vi "CheckTemplateChange.vi"(8 "Template #":i8, 9 "Template":string, 10 "Settings In":T1={"Name of test"="", "Date"=timestamp(0 s since 1904-01-01), "Location"="", "Template"="", "Soundcard"="", "resolution"=0, "Sampling rate"=0, "Ch1 Gain "=0.0, "Ch2 Gain"=0.0, "Sample time (s)"=0.0, "Pre-trigger (s)"=0.0, "Hammer Threshold"=0.0, "Positions"=0, "Taps/Position"=0, "Set Names"="", "Freq resolution"=0.0, "Hammer cutoff"=0.0, "Mic cutoff"=0.0, "Double bounce "=0.0, "Hammer Cal"=0.0, "dB Offset"=0.0, "Accel Cal"=0.0, "Vibrometer Cal"=0.0, "Mic Cal"=0.0, "Output"=0, "Voltage Cal"=0.0, "Vibrometer Port"="", "Range"=0, "High Pass"=0, "Bandwidth"=0, "X Range"=[], "Y Range"=[], "dB Spread"=0.0, "Trigger"=0, "Ch_1"=0, "Ch_2"=0, "flip?"=FALSE, "60Hz"=FALSE, "Time offset"=0.0, "Piezo Cal"=1.0, "Default Notes"=""} {"Ch_2" min=1 step=1; "Ch_1" min=1 max=100 step=1; "Trigger" items=["Hammer (force)", "Self-tap", "Spacebar"]; "Bandwidth" items=["1 kHz"=1, "5 kHz"=5, "10 kHz"=10, "25 kHz"=25, "50 kHz"=50, "100 kHz"=100]; "High Pass" items=["Off", "13 Hz", "104 Hz"]; "Range" items=["10 mm/s"=1, "20 mm/s"=2, "50 mm/s"=5, "100 mm/s"=10, "200 mm/s"=20, "500 mm/s"=50, "1 m/s"=100, "2 m/s"=200]; "Output" items=["Accelerometer", "Speed (from acceleration)", "Microphone", "Vibrometer", "Piezo"]; "Voltage Cal" format="%#_13g"; "Ch2 Gain" format="%#_13g"; "Ch1 Gain" format="%#_13g"; "Double bounce" min=0.0; "Mic cutoff" min=0.0 format="%#_4g"; "Hammer cutoff" min=0.0 format="%#_4g"; "Freq resolution" min=0.0; "Pre-trigger (s)" format="%#_13g"; "Date" format="%<%H:%M\n%d/%m/%y>T"; "resolution" items=["16 bit"=16, "24 bit"=24, "32 bit"=32]; "Sampling rate" items=["22050 samp/s"=22050, "44100 samp/s"=44100, "48000 samp/s"=48000]}, 11 "Path To Instrument Folder":path) -> (2 "Template":u16, 3 "Settings  Out":T1={"Name of test"="", "Date"=timestamp(0 s since 1904-01-01), "Location"="", "Template"="", "Soundcard"="", "resolution"=0, "Sampling rate"=0, "Ch1 Gain "=0.0, "Ch2 Gain"=0.0, "Sample time (s)"=0.0, "Pre-trigger (s)"=0.0, "Hammer Threshold"=0.0, "Positions"=0, "Taps/Position"=0, "Set Names"="", "Freq resolution"=0.0, "Hammer cutoff"=0.0, "Mic cutoff"=0.0, "Double bounce "=0.0, "Hammer Cal"=0.0, "dB Offset"=0.0, "Accel Cal"=0.0, "Vibrometer Cal"=0.0, "Mic Cal"=0.0, "Output"=0, "Voltage Cal"=0.0, "Vibrometer Port"="", "Range"=0, "High Pass"=0, "Bandwidth"=0, "X Range"=[], "Y Range"=[], "dB Spread"=0.0, "Trigger"=0, "Ch_1"=0, "Ch_2"=0, "flip?"=FALSE, "60Hz"=FALSE, "Time offset"=0.0, "Piezo Cal"=1.0, "Default Notes"=""} {"Ch_2" min=1 step=1; "Ch_1" min=1 max=100 step=1; "Trigger" items=["Hammer (force)", "Self-tap", "Spacebar"]; "Bandwidth" items=["1 kHz"=1, "5 kHz"=5, "10 kHz"=10, "25 kHz"=25, "50 kHz"=50, "100 kHz"=100]; "High Pass" items=["Off", "13 Hz", "104 Hz"]; "Range" items=["10 mm/s"=1, "20 mm/s"=2, "50 mm/s"=5, "100 mm/s"=10, "200 mm/s"=20, "500 mm/s"=50, "1 m/s"=100, "2 m/s"=200]; "Output" items=["Accelerometer", "Speed (from acceleration)", "Microphone", "Vibrometer", "Piezo"]; "Voltage Cal" format="%#_13g"; "Ch2 Gain" format="%#_13g"; "Ch1 Gain" format="%#_13g"; "Double bounce" min=0.0; "Mic cutoff" min=0.0 format="%#_4g"; "Hammer cutoff" min=0.0 format="%#_4g"; "Freq resolution" min=0.0; "Pre-trigger (s)" format="%#_13g"; "Date" format="%<%H:%M\n%d/%m/%y>T"; "resolution" items=["16 bit"=16, "24 bit"=24, "32 bit"=32]; "Sampling rate" items=["22050 samp/s"=22050, "44100 samp/s"=44100, "48000 samp/s"=48000]})   [LabVIEW 2022 SP3]
uses:
  PreferencesControl.ctl
panel:
  # "Hz"
  # "dB"
  # "dB"
  # "sec"
  # "sec"
  # "mV/Pa"
  # "mV/m/s2"
  # "mV/mm/s"
  # "V/N"
  # "sec"
  # "sec"
  # "mV/N"
  # "a.u."
  # "a.u."
  # "sec"
  # "Hz"
  # "dB"
  # "dB"
  # "sec"
  # "sec"
  # "mV/Pa"
  # "mV/m/s2"
  # "mV/mm/s"
  # "V/N"
  # "sec"
  # "sec"
  # "mV/N"
  # "a.u."
  # "a.u."
  # "sec"
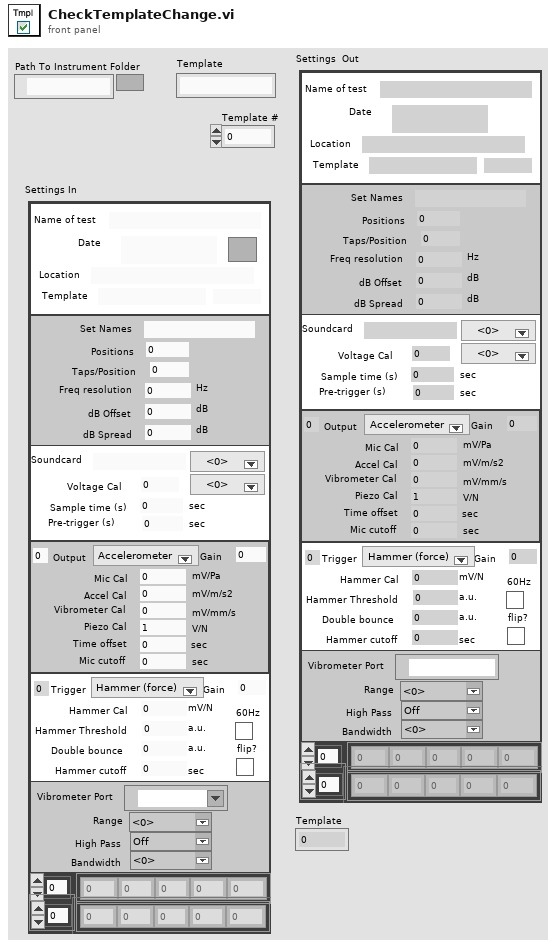
[diagram p1: front panel]
types:
  T1 = typedef "PreferencesControl.ctl" = cluster{"Name of test":string, "Date":timestamp, "Location":string, "Template":string, "Soundcard":string, "resolution":u16, "Sampling rate":u16, "Ch1 Gain ":dbl, "Ch2 Gain":dbl, "Sample time (s)":dbl, "Pre-trigger (s)":dbl, "Hammer Threshold":dbl, "Positions":i16, "Taps/Position":i16, "Set Names":string, "Freq resolution":dbl, "Hammer cutoff":dbl, "Mic cutoff":dbl, "Double bounce ":dbl, "Hammer Cal":dbl, "dB Offset":dbl, "Accel Cal":dbl, "Vibrometer Cal":dbl, "Mic Cal":dbl, "Output":u16, "Voltage Cal":dbl, "Vibrometer Port":refnum<visa-resource-name>, "Range":u16, "High Pass":u16, "Bandwidth":u16, "X Range":cluster{"Minimum":dbl, "Maximum":dbl, "Increment":dbl, "Minor Increment":dbl, "Start":dbl}[], "Y Range":cluster{"Minimum":dbl, "Maximum":dbl, "Increment":dbl, "Minor Increment":dbl, "Start":dbl}[], "dB Spread":dbl, "Trigger":u16, "Ch_1":u8, "Ch_2":u8, "flip?":bool, "60Hz":bool, "Time offset":dbl, "Piezo Cal":dbl, "Default Notes":string}
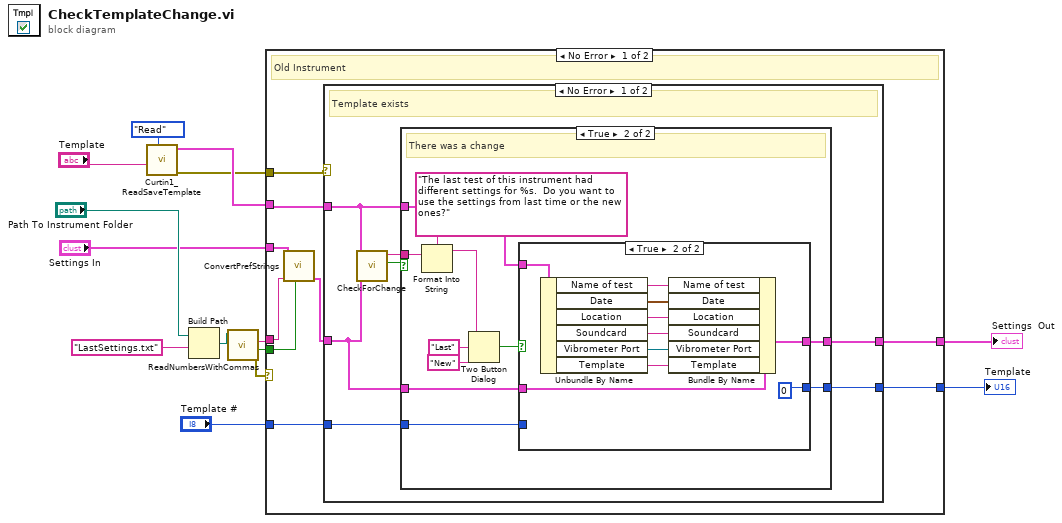
[diagram p0: block diagram]
diagram:
  n1 = call "Curtin1_ReadSaveTemplate.vi"("Task"=enum16{"Save", "Read", "List"}."Read", "Template"="Template") -> ("error out"=w5:errorcluster, "Settings out"=w6:T1)  [unwired: 6 in, 2 out]
  n2 = Build Path(base path="Path To Instrument Folder", name or relative path="LastSettings.txt") -> (appended path=w4:path)
  n3 = call "ReadNumbersWithCommas.vi"("file (use dialog)"=w4) -> ("error out"=w3:errorcluster, "comma?"=w1:bool, "text"=w2:string)  [unwired: 7 in, 1 out]
  n4 = case shown="No Error" w3 {
    tunnel: w2 -> [w23 _]
    tunnel: "Settings In" -> [w22 _]
    tunnel: [w19 w58] -> w11
    tunnel: w6 -> [w18 w59]
    tunnel: "Template #" -> [w17 w58]
    tunnel: [w21 w59] -> w8
    tunnel: w5 -> [w16 _]
    tunnel: w1 -> [w15 _]
    frame No Error {
      # "Old Instrument"
      n5 = call "ConvertPrefStrings.vi"("Comma?"=w15, "String In"=w23, "Settings"=w22) -> ("Settings"=w20:T1)  [unwired: 7 in, 1 out]
      n6 = case shown="No Error" w16 {
        tunnel: [w28 w56] -> w21
        tunnel: w20 -> [w27 w56]
        tunnel: [w26 w57] -> w19
        tunnel: w18 -> [w25 _]
        tunnel: w17 -> [w24 w57]
        frame No Error {
          # "Template exists"
          n7 = call "CheckForChange.vi"("Original Settings"=w27, "Current Settings"=w25) -> ("change?"=w30:bool, "list of changes"=w29:string)  [unwired: 8 in]
          n8 = case shown="True" w30 {
            tunnel: w29 -> [_ w42]
            tunnel: [w32 w37] -> w28
            tunnel: w27 -> [_ w36]
            tunnel: [w31 w35] -> w26
            tunnel: w25 -> [w32 w34]
            tunnel: w24 -> [w31 w33]
            frame False {
              # "Same settings"
            }
            frame True {
              # "There was a change"
              n9 = Format Into String(format string="The last test of this instrument had different settings for %s.  Do you want to use the settings from last time or the new ones?", w42) -> (resulting string=w41:string)  [unwired: 2 in, 1 out]
              n10 = Two Button Dialog(message=w41, 1:"New" ("F button name (\"Cancel\")"), 2:"Last" ("T button name (\"OK\")")) -> (T button?=w38:bool)
              n11 = case shown="True" w38 {
                tunnel: [w45 w47] -> w37
                tunnel: w36 -> [_ w48]
                tunnel: [w44 0] -> w35
                tunnel: w34 -> [w45 w49]
                tunnel: w33 -> [w44 _]
                frame False {
                }
                frame True {
                  n12 = Unbundle By Name(w49) -> ("Name of test"=w54:string, "Date"=w53:timestamp, "Location"=w52:string, "Soundcard"=w51:string, "Vibrometer Port"=w50:refnum<visa-resource-name>, "Template"=w46:string)
                  n13 = Bundle By Name(cluster=w48, "Name of test"=w54, "Date"=w53, "Location"=w52, "Soundcard"=w51, "Vibrometer Port"=w50, "Template"=w46) -> (w47:T1)
                }
              }
            }
          }
        }
        frame Error {
          # "Template selection does not exist"
        }
      }
    }
    frame Error {
      # "New Instrument"
    }
  }
  "Template" <- w11
  "Settings  Out" <- w8
